vi "DataInsert.vi"() -> ()   [LabVIEW 2024]
uses:
  <vilib>/addons/database/Connection.llb/DB Tools Open Connec (Path).vi
  <vilib>/addons/database/NI_Database_API.lvlib
panel:
  in  "DataInsert":cluster{"ID":string, "Grade":dbl, "Age":dbl}[](array[cluster])
  in  "connection information":path
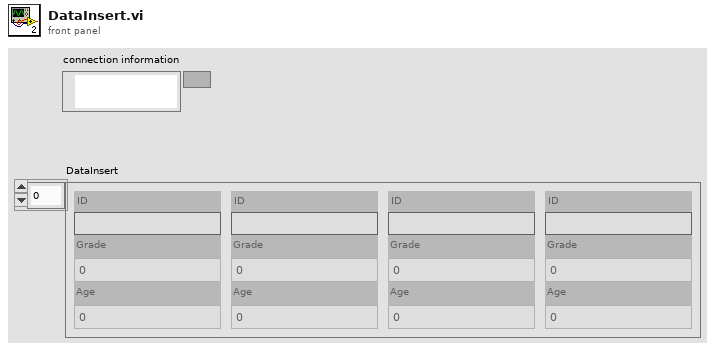
[diagram p1: front panel]
types:
  T1 = typedef "NI_Database_API.lvlib/Conn ObjectReference.ctl" = refnum<k1>
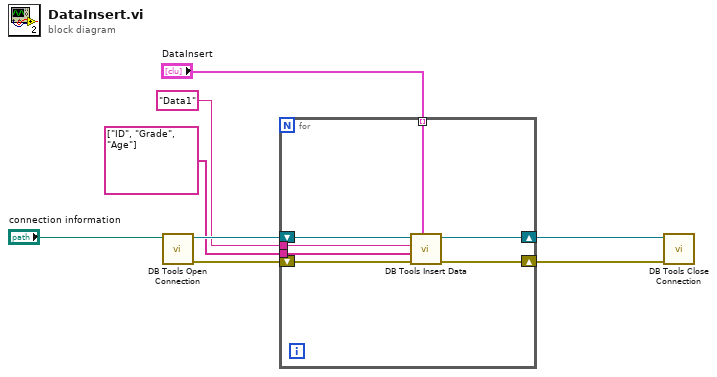
[diagram p0: block diagram]
diagram:
  n1 = call-poly <vilib>:"DB Tools Open Connection.vi"("connection information"="connection information") -> ("error out"=w4:errorcluster, "connection reference"=w7:T1)  [unwired: 7 in]
  n2 = for {
    tunnel: "Data1" ("table") -> [w11]
    tunnel: string[] ["ID", "Grade", "Age"] ("columns") -> [w10]
    tunnel: "DataInsert" -> [w9] mode=indexing
    shift-right: [w14] -> w6
    shift-left: w7 -> [w15]
    shift-right: [w13] -> w5
    shift-left: w4 -> [w12]
    n3 = call <vilib>:"DB Tools Insert Data.vi"("data"=w9, "error in (no error)"=w12, "columns"=w10, "table"=w11, "connection reference"=w15) -> ("error out"=w13:errorcluster, "connection reference out"=w14:T1)  [unwired: 5 in]
  }
  n4 = call <vilib>:"DB Tools Close Connection.vi"("error in (no error)"=w5, "connection reference"=w6) -> ()  [unwired: 5 in, 1 out]
